vi "CalcKnee.vi"(2 "Voltage":dbl[](array[numeric]), 3 "Power":dbl[](array[numeric]), 4 "Current":dbl[](array[numeric])) -> (0 "Knee Voltage":dbl, 1 "Knee Current":dbl)   [LabVIEW 2012, in "Instruments.lvclass"]
uses:
  Instruments.lvclass
  <vilib>/Analysis/6fits.llb/Curve Fitting Criteria.ctl
  <vilib>/Analysis/NI_AALPro.lvlib
  <vilib>/gmath/NI_Gmath.lvlib
panel:
  out "xi used":dbl[](array[numeric]) format="%_6g"
  out "yi":dbl[](array[numeric]) format="%_6g"
  in  "transposed array":dbl[][](array[numeric])=[[1.0, 6.1583, 18.199999999999996, 279.4207352341019], [2.0, 7.0202, 48.69999999999998, 279.0471941984746], [5.0, 9.0886, 140.86666666666667, 278.3000100182607], [10.0, 11.6588, 282.0999999999999, 278.3000100182607], [15.0, 13.571, 417.76666666666665, 277.9263668963827], [20.0, 15.136, 545.7666666666667, 277.9263668963827], [25.0, 16.537, 669.4333333333333, 278.3000100182607], [30.0, 17.834, 790.1, 278.3000100182607], [35.0, 19.055, 907.7666666666668, 278.3000100182607], [40.0, 20.223, 1022.1, 278.3000100182607], [45.0, 21.344, 1133.1, 278.3000100182607], [50.0, 22.437, 1242.1, 278.3000100182607]]
  out "Best Linear Fit":dbl[](array[numeric])
  out "XY Graph":cluster{"all rows":dbl[], "all rows":dbl[]}(graph)
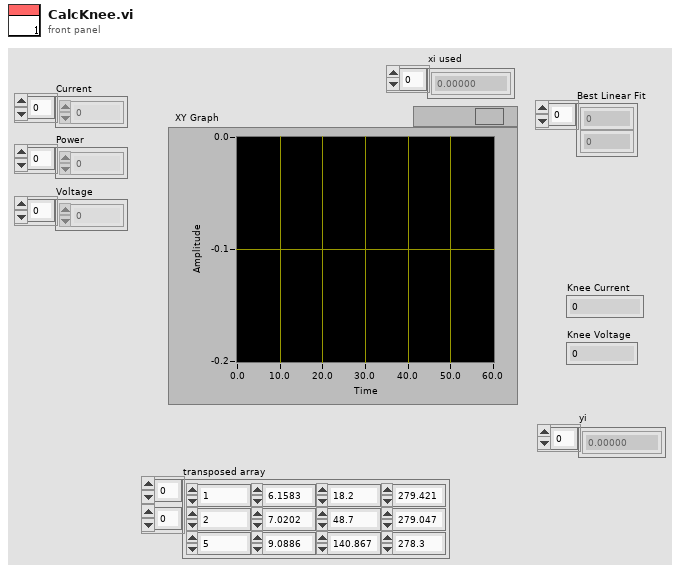
[diagram p1: front panel]
types:
  T1 = typedef "NI_AALPro.lvlib/Curve Fitting Criteria.ctl" = u16
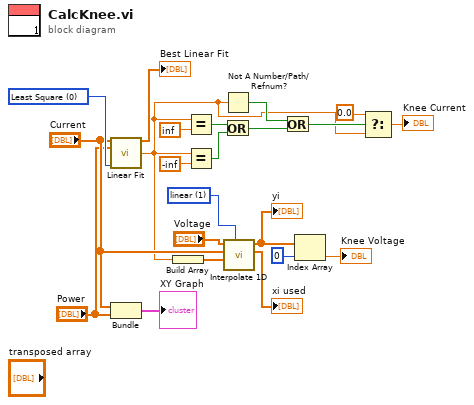
[diagram p0: block diagram]
diagram:
  w18 = 1 items=["nearest", "linear", "spline", "cubic Hermite", "Lagrange"] ("method")
  w21 = T1 0 items=["Least Square", "Least Absolute Residual", "Bisquare"] ("method")
  n1 = call <vilib>:"Linear Fit.vi"("Y"="Current", "X"="Power", "method"=w21) -> ("Best Linear Fit"=→"Best Linear Fit":dbl[], "intercept"=w5:dbl)  [unwired: 8 in, 3 out]
  n2 = Bundle("Current"="Current", "Power"="Power") -> (→"XY Graph":cluster{"Current":dbl[], "Power":dbl[]})  [unwired: 1 in]
  n3 = Build Array(w5) -> (w19:dbl[])
  n4 = Equal?(x=w5, y=inf) -> (x = y?=w2:bool)
  n5 = Equal?(x=w5, y=-inf) -> (x = y?=w8:bool)
  n6 = Not A Number/Path/Refnum?(number/path/refnum=w5) -> (NaN/Path/Refnum?=w7:bool)
  n7 = Or(x=w2, y=w8) -> (x .or. y?=w1:bool)
  n8 = call <vilib>:"Interpolate 1D.vi"("method"=w18, "xi"=w19, "X"="Current", "Y"="Voltage") -> ("xi used"=→"xi used":dbl[], "yi"=w17:dbl[])  [unwired: 5 in, 1 out]
  "yi" <- w17
  n9 = Or(x=w7, y=w1) -> (x .or. y?=w6:bool)
  n10 = Index Array(array=w17, index=0) -> (element=→"Knee Voltage":dbl)
  n11 = Select(t=0.0, s=w6, f=w5) -> (s? t:f=→"Knee Current":dbl)
